vi "Launch.vi"   [LabVIEW 2022 SP3]
uses:
  Components/ViPER.lvlibp/ViPER.lvclass
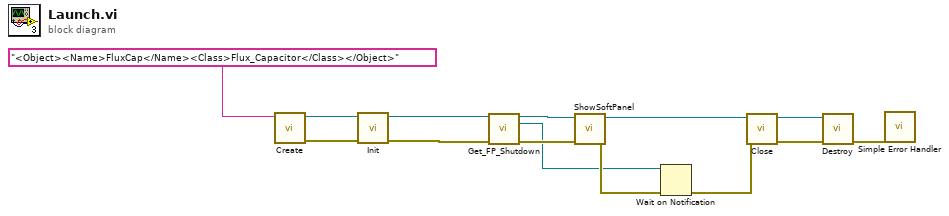
[diagram p0: block diagram]
diagram:
  n1 = call "Create.vi"("Config XML"="<Object><Name>FluxCap</Name><Class>Flux_Capacitor</Class></Object>") -> ("error out"=w4:errorcluster, "reference out"=w14:refnum<class "ViPER.lvclass">)  [unwired: 9 in]
  n2 = call-dynamic "Init.vi"("error in (no error)"=w4, "reference in"=w14) -> ("error out"=w9:errorcluster, "reference out"=w10:refnum<class "ViPER.lvclass">)  [unwired: 8 in]
  n3 = call "Get_FP_Shutdown.vi"("ViPER_Base in"=w10, "error in (no error)"=w9) -> ("ViPER_Base out"=w7:refnum<class "ViPER.lvclass">, "SoftFP_Shutdown"=w5:refnum<notifier>, "error out"=w8:errorcluster)  [unwired: 10 in, 1 out]
  n4 = call-dynamic "ShowSoftPanel.vi"("error in (no error)"=w8, "Driver in"=w7) -> ("error out"=w6:errorcluster, "Driver out"=w2:refnum<class "ViPER.lvclass">)  [unwired: 7 in, 1 out]
  n5 = Wait on Notification(notifier=w5, error in (no error)=w6) -> (error out=w3:errorcluster)  [unwired: 2 in, 3 out]
  n6 = call-dynamic "Close.vi"("error in (no error)"=w3, "reference in"=w2) -> ("error out"=w12:errorcluster, "reference out"=w13:refnum<class "ViPER.lvclass">)  [unwired: 8 in]
  n7 = call "Destroy.vi"("error in (no error)"=w12, "reference in"=w13) -> ("error out"=w1:errorcluster)  [unwired: 9 in]
  n8 = call <vilib>:"Simple Error Handler.vi"("error in (no error)"=w1) -> ()  [unwired: 4 in, 5 out]
